vi "CreateArray.vi"(8 "error in (no error)":errorcluster, 9 "ChildType":refnum<class "LVType.lvclass">, 10 "Dimension":u32=1, 11 "ID":string) -> (0 "error out":errorcluster, 3 "LVArrayType out":refnum<class "LVArrayType.lvclass">)   [LabVIEW 2020, in "LVDataTypes.lvlib" / "LVArrayType.lvclass"]
uses:
  <vilib>/AppBuilder/Engine/WebServiceDescription/LVDataTypes/LVArrayType/LVArrayType.lvclass
  e:/builds/penguin/labview/branches/2020/dev/dist/vi.lib/AppBuilder/Engine/WebServiceDescription/LVDataTypes/LVType/LVType.lvclass
  <vilib>/AppBuilder/Engine/WebServiceDescription/LVDataTypes/LVType/LVType.lvclass
  <vilib>/AppBuilder/Engine/WebServiceDescription/LVDataTypes/TypeCode.ctl
  <vilib>/AppBuilder/Engine/WebServiceDescription/LVDataTypes/LVArrayType/LVArrayType.lvclass/LVArrayType.ctl
  <vilib>/AppBuilder/Engine/WebServiceDescription/LVDataTypes/LVDataTypes.lvlib
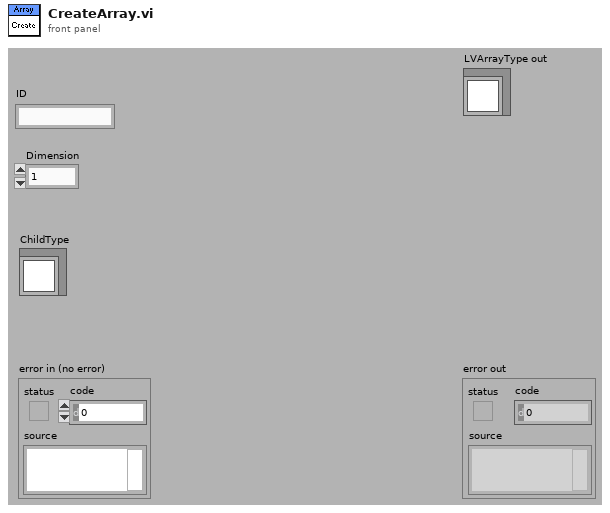
[diagram p1: front panel]
types:
  T1 = typedef "LVDataTypes.lvlib/TypeCode.ctl" = enum16{"Undefined", "Byte", "Unsigned Byte", "Word", "Unsigned Word", "Long", "Unsigned Long", "Quad", "Unsigned Quad", "Single", "Double", "Extended", "Enum", "Boolean", "String", "Path", "Array", "Cluster", "AnalogWaveform", "DigitalWaveform", "Time Stamp", "Void", "Complex Single", "Complex Double", "Complex Extended"}
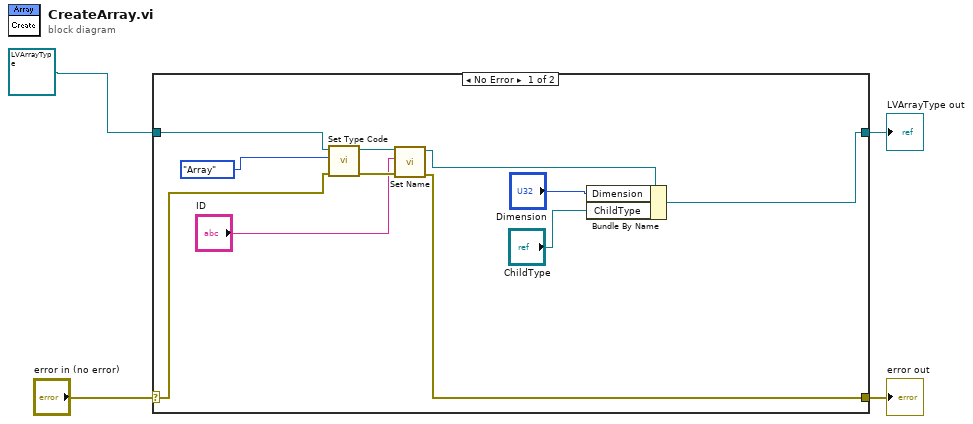
[diagram p0: block diagram]
diagram:
  n1 = case shown="No Error" "error in (no error)" {
    selector: "error in (no error)" -> [w9 w17]
    tunnel: [w6 w17] -> w3
    tunnel: [w13 w16] -> w2
    tunnel: refnum<class "LVArrayType.lvclass"> refnum ("LVDataTypes.lvlib:LVArrayType.lvclass") -> [w5 w16]
    frame No Error {
      n2 = call <vilib>:"Set Type Code.vi"("error in (no error)"=w9, "Type"=TypeCode."Array", "LVType.lvclass in"=w5) -> ("error out"=w11:errorcluster, "LVType.lvclass out"=w12:refnum<class "LVArrayType.lvclass">)  [unwired: 7 out]
      n3 = call <vilib>:"Set Name.vi"("error in (no error)"=w11, "Name"="ID", "LVType.lvclass in"=w12) -> ("error out"=w6:errorcluster, "LVType.lvclass out"=w7:refnum<class "LVArrayType.lvclass">)  [unwired: 7 out]
      n4 = Bundle By Name(cluster=w7, "Dimension"="Dimension", "ChildType"="ChildType") -> (w13:refnum<class "LVArrayType.lvclass">)
    }
    frame Error {
    }
  }
  "error out" <- w3
  "LVArrayType out" <- w2
